vi "CH_LM Config Tune Zoom.vi"(0 "Meter Index":i32, 1 "Display Mode":bool, 2 "Direction (horizontal)":bool, 3 "Zoom Mode (1)":T1=enum."1", 5 "error in (no error)":errorcluster, 7 "Timeout / ms (3000)":i32=1000, 8 "Action (query)":bool, 9 "Lock Timeout / ms (1000)":i32=1000) -> (11 "Lock timed out":bool, 14 "Meter Index":i32, 17 "Zoom Mode":T1=enum."1", 19 "error out":errorcluster)   [LabVIEW 2012, in "CH_LM.lvlib"]
doc: "This command will set/query the trend zoom mode when in Strip Chart or Bar Chart mode."
uses:
  CH_LM.lvlib
  CH_LM Zoom Factor.ctl
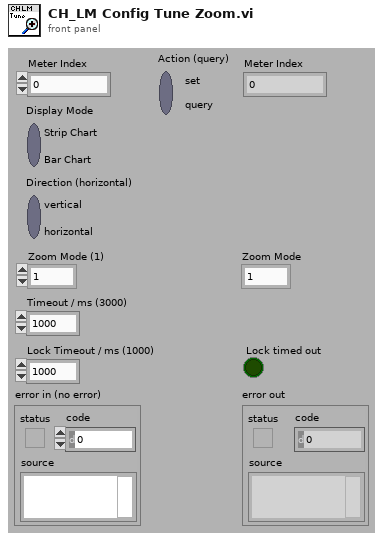
[diagram p1: front panel]
types:
  T1 = typedef "CH_LM.lvlib/CH_LM Zoom Factor.ctl" = enum16{"Auto", "1", "2", "5", "10", "20"}
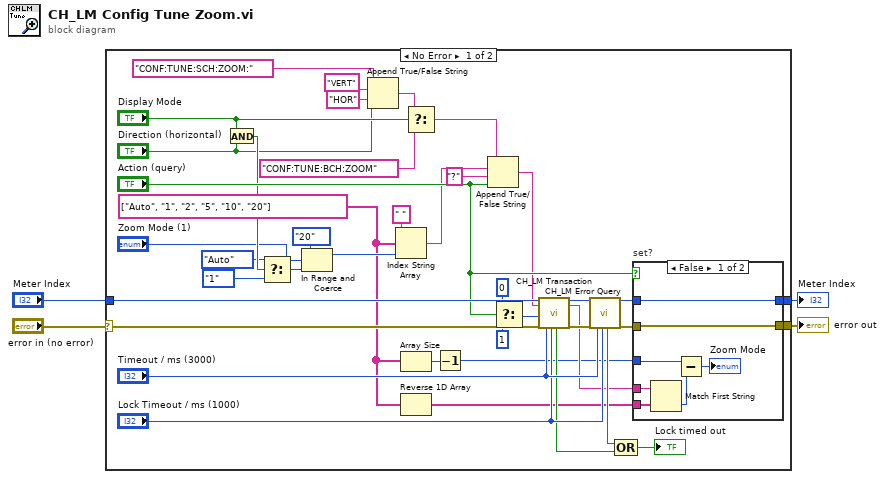
[diagram p0: block diagram]
diagram:
  n1 = case shown="No Error" "error in (no error)" {
    selector: "error in (no error)" -> [w45 w56]
    tunnel: [w43 w56] -> w4
    tunnel: "Meter Index" -> [w44 w55]
    tunnel: [w42 w55] -> w1
    frame No Error {
      w8 = string[] ["Auto", "1", "2", "5", "10", "20"]
      n2 = And(x="Display Mode", y="Direction (horizontal)") -> (x .and. y?=w26:bool)
      n3 = Select(t=enum16{"Auto", "1", "2", "5", "10", "20"}."Auto" ("lower limit"), s=w26, f=enum16{"Auto", "1", "2", "5", "10", "20"}."1") -> (s? t:f=w25:enum16{"Auto", "1", "2", "5", "10", "20"})
      n4 = In Range and Coerce(upper limit=enum16{"Auto", "1", "2", "5", "10", "20"}."20", x="Zoom Mode (1)", lower limit=w25) -> (coerced(x)=w27:T1)  [unwired: 1 out]
      n5 = Append True/False String(1:"Direction (horizontal)", 2:"HOR" ("false string"), 3:"VERT" ("true string"), 4:"CONF:TUNE:SCH:ZOOM:" ("Command String")) -> (0:w13:string)
      n6 = Index String Array(1:w27, 2:w8, 3:" " ("string (\"\")")) -> (0:w22:string)
      n7 = Array Size(array=w8) -> (size(s)=w7:i32)
      n8 = Reverse 1D Array(array=w8) -> (reversed array=w5:string[])
      n9 = Select(t=w13, s="Display Mode", f="CONF:TUNE:BCH:ZOOM" ("Command String")) -> (s? t:f=w19:string)
      n10 = Decrement(x=w7) -> (x-1=w6:i32)
      n11 = Append True/False String(1:"Action (query)", 2:"?" ("true string"), 3:w22, 4:w19) -> (0:w21:string)
      n12 = Select(t=0, s="Action (query)", f=1 ("NofStrings (-1:all)")) -> (s? t:f=w29:i32)
      n13 = call "CH_LM Transaction.vi"("Meter Index"=w44, "Command String"=w21, "NofStrings (-1:all)"=w29, "error in (no error)"=w45, "Timeout / ms (3000)"="Timeout / ms (3000)", "Lock Timeout / ms (1000)"="Lock Timeout / ms (1000)") -> ("Lock timed out"=w33:bool, "Meter Index"=w12:i32, "Response"=w10:string, "error out"=w11:errorcluster)  [unwired: 10 out]
      n14 = call "CH_LM Error Query.vi"("Meter Index"=w12, "error in (no error)"=w11, "Timeout / ms (3000)"="Timeout / ms (3000)", "Lock Timeout / ms (1000)"="Lock Timeout / ms (1000)") -> ("Lock timed out"=w34:bool, "Meter Index"=w36:i32, "error out"=w35:errorcluster)  [unwired: 13 out]
      n15 = Compound Arithmetic op=OR(w34, w33) -> (→"Lock timed out":bool)
      n16 = case "set?" shown="False" "Action (query)" {
        tunnel: w35 -> [w51 w54]
        tunnel: [w51 w54] -> w43
        tunnel: w36 -> [w52 w53]
        tunnel: [w52 w53] -> w42
        tunnel: w10 -> [w50 _]
        tunnel: w5 -> [w49 _]
        tunnel: w6 -> [w48 _]
        frame False {
          n17 = Match First String(2:w49, 3:w50) -> (0:w47:i32)  [unwired: 1 out]
          n18 = Subtract(x=w48, y=w47) -> (x-y=→"Zoom Mode":i32)
        }
        frame True {
        }
      }
    }
    frame Error {
    }
  }
  "error out" <- w4
  "Meter Index" <- w1
